vi "Lift Teleop.vi"(11 "Cluster":T1={"Axes Right"=[0.031496062992125984, 0.0, 0.984251968503937], " Axes Left"=[0.05511811023622047, 0.0, -1.0], " Axes Co-driver"=[-0.023622047244094488, -0.015748031496062992, 0.0, 0.0, 0.047244094488188976, -0.031496062992125984], "Buttons Right"=[FALSE, FALSE, FALSE, FALSE, FALSE, FALSE, FALSE, FALSE, FALSE, FALSE, FALSE], "Buttons Left"=[FALSE, FALSE, FALSE, FALSE, FALSE, FALSE, FALSE, FALSE, FALSE, FALSE, FALSE], "Buttons Co-driver"=[FALSE, FALSE, FALSE, FALSE, FALSE, FALSE, FALSE, FALSE, FALSE, FALSE], "POVs Right"=[], "POVs Left"=[], "POVs Co-driver"=[-1]}) -> ()   [LabVIEW 2016]
uses:
  Joystick vals.ctl
  <vilib>/Rock Robotics/Network Tables/NT Read Number.vi
panel:
  in  "Output":dbl=1.0
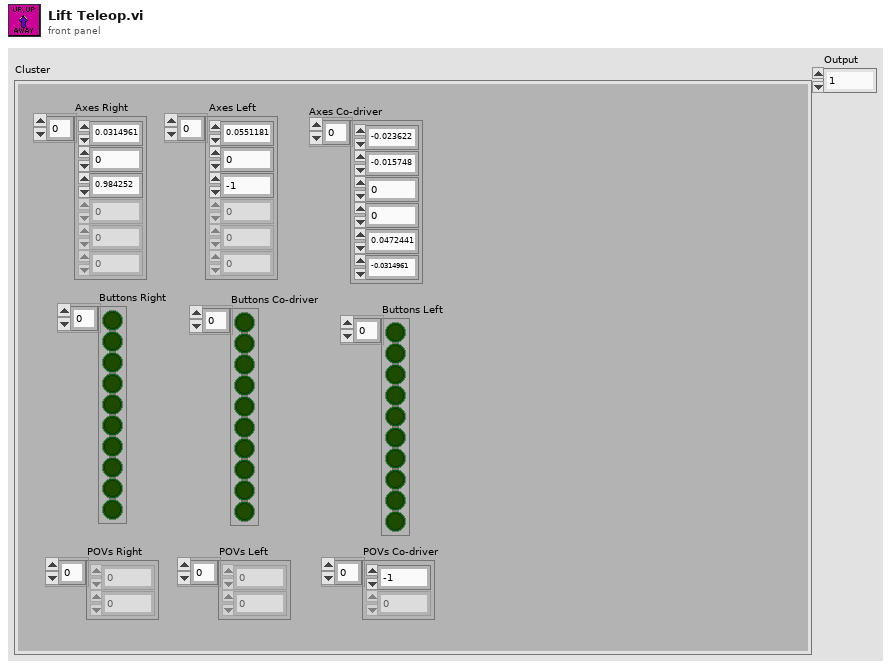
[diagram p1: front panel]
types:
  T1 = typedef "Joystick vals.ctl" = cluster{"Axes Right":dbl[], " Axes Left":dbl[], " Axes Co-driver":dbl[], "Buttons Right":bool[], "Buttons Left":bool[], "Buttons Co-driver":bool[], "POVs Right":i16[], "POVs Left":i16[], "POVs Co-driver":i16[]}
  T2 = typedef "WPI_MotorControlDeviceRef.ctl" = cluster{"DeviceStatus":errorcluster, "Type":T3, "PWM":cluster{"PWM Channel":T4, "DeadBand":T5}, "CAN":cluster{"Device Number":u8, "SetOutput VI Ref":variant, "GetOutput VI Ref":variant, "Enable VI Ref":variant, "Disable VI Ref":variant, "Data":variant}, "Invert":bool}
  T3 = typedef "WPI_MotorControlType.ctl" = enum16{"PWM", "CAN"}
  T4 = typedef "FPGA_DIOPWMChannel.ctl" = enum8{"PWM 0", "PWM 1", "PWM 2", "PWM 3", "PWM 4", "PWM 5", "PWM 6", "PWM 7", "PWM 8", "PWM 9", "PWM MXP 0", "PWM MXP 1", "PWM MXP 2", "PWM MXP 3", "PWM MXP 4", "PWM MXP 5", "PWM MXP 6", "PWM MXP 7", "PWM MXP 8", "PWM MXP 9", "Invalid"}
  T5 = typedef "WPI_PWMDeadband.ctl" = cluster{"Name":string, "maxPositivePwm":i32, "minPositivePwm":i32, "centerPwm":i32, "maxNegativePwm":i32, "minNegativePwm":i32, "angularRange":u16}
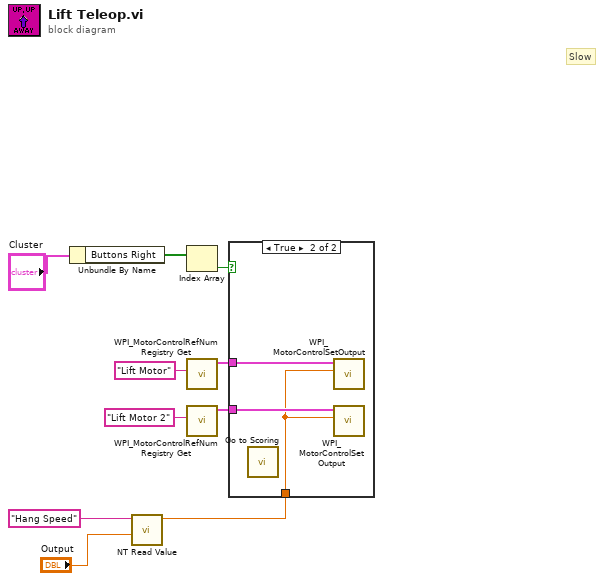
[diagram p0: block diagram]
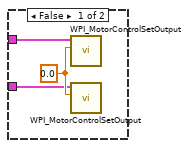
[diagram p2: hidden frame]
diagram:
  # "Slow"
  n1 = Unbundle By Name("Cluster") -> ("Buttons Right"=w3:bool[])
  n2 = call-poly <vilib>:"NT Read Value.vi"("Default Value"="Output", "Name"="Hang Speed") -> ("Numeric"=w1:dbl)  [unwired: 8 in, 1 out]
  n3 = Index Array(array=w3) -> (element=w2:bool)  [unwired: 1 in]
  n4 = call <vilib>:"WPI_MotorControlRefNum Registry Get.vi"("refnum name"="Lift Motor") -> ("MotorControlDevRef"=w8:T2)  [unwired: 9 in, 1 out]
  n5 = call <vilib>:"WPI_MotorControlRefNum Registry Get.vi"("refnum name"="Lift Motor 2") -> ("MotorControlDevRef"=w4:T2)  [unwired: 9 in, 1 out]
  n6 = case shown="True" w2 {
    tunnel: w8 -> [w12 w16]
    tunnel: w4 -> [w11 w15]
    tunnel: w1 -> [_ w14]
    frame False {
      w13 = 0.0 ("Output 2")
      n7 = call <vilib>:"WPI_MotorControlSetOutput.vi"("Output"=w13, "MotorControlDevRef"=w12) -> ()  [unwired: 7 in, 3 out]
      n8 = call <vilib>:"WPI_MotorControlSetOutput.vi"("Output"=w13, "MotorControlDevRef"=w11) -> ()  [unwired: 7 in, 3 out]
    }
    frame True {
      n9 = call "Go to Scoring.vi"() -> ()  [unwired: 11 in, 1 out]
      n10 = call <vilib>:"WPI_MotorControlSetOutput.vi"("Output"=w14, "MotorControlDevRef"=w16) -> ()  [unwired: 7 in, 3 out]
      n11 = call <vilib>:"WPI_MotorControlSetOutput.vi"("Output"=w14, "MotorControlDevRef"=w15) -> ()  [unwired: 7 in, 3 out]
    }
  }
